vi "Escape JSON.vi"(11 "JSON":string) -> (3 "Escaped JSON":string)   [LabVIEW 2015, in "NI_JSON Parsing.lvlib"]
uses:
  NI_JSON Parsing.lvlib
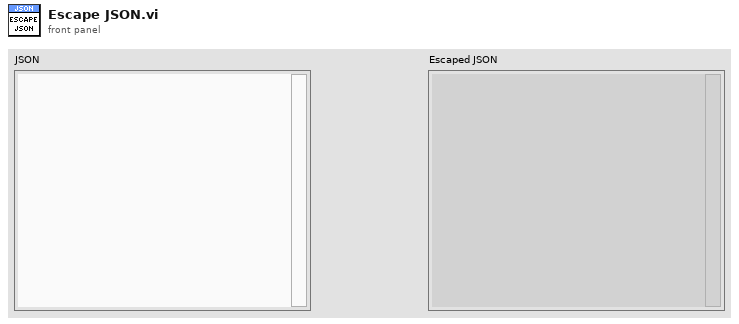
[diagram p1: front panel]
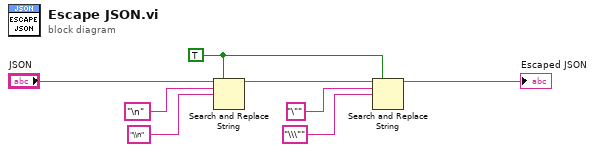
[diagram p0: block diagram]
diagram:
  w7 = TRUE ("replace all? (F)")
  n1 = Search and Replace String(replace all?=w7, input string="JSON", search string="\n", replace string="\\n") -> (result string=w8:string)  [unwired: 4 in, 3 out]
  n2 = Search and Replace String(replace all?=w7, input string=w8, search string="\"", replace string="\\\"") -> (result string=→"Escaped JSON":string)  [unwired: 4 in, 3 out]
